vi "Main.vi"() -> ()   [LabVIEW 2023]
panel:
  out "Result":dbl
  in  "Divide":bool
  in  "Multiply":bool
  in  "Subtract":bool
  in  "Add":bool
  in  "Operand 2":dbl
  in  "Operand 1":dbl
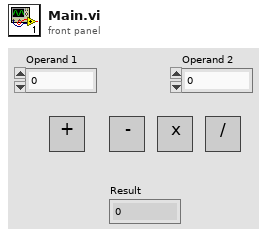
[diagram p1: front panel]
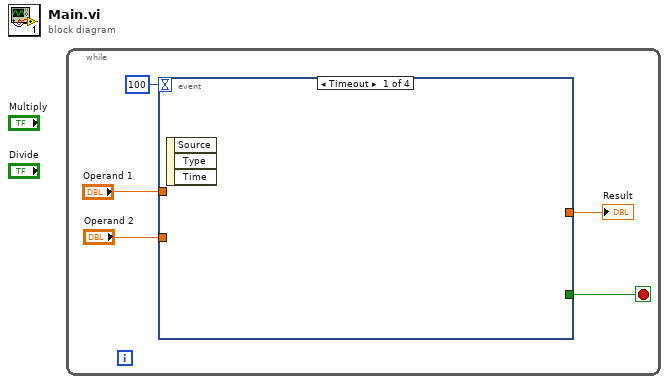
[diagram p0: block diagram]
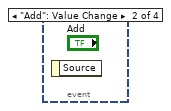
[diagram p2: hidden frame]
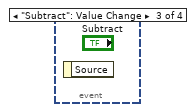
[diagram p3: hidden frame]
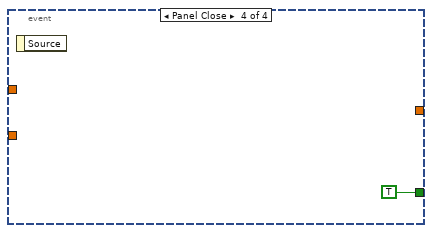
[diagram p4: hidden frame]
diagram:
  n1 = while {
    stop <- w1 stop-if-true
    n2 = event shown="[0] Timeout" {
      selector: _ -> [_ _ _ _]
      dyn-events: _ -> [_ _ _ _]
      timeout: 100 -> [_ _ _ _]
      tunnel: "Operand 1" -> [_ _ _ _]
      tunnel: "Operand 2" -> [_ _ _ _]
      tunnel: [_ _ _ _] -> w2
      tunnel: [_ _ _ TRUE] -> w1
      event Timeout {
        n3 = event-data() -> ()  [unwired: 1 in, 3 out]
      }
      event "Add": Value Change {
        n4 = event-data() -> ()  [unwired: 1 in, 1 out]
      }
      event "Subtract": Value Change {
        n5 = event-data() -> ()  [unwired: 1 in, 1 out]
      }
      event Panel Close {
        n6 = event-data() -> ()  [unwired: 1 in, 1 out]
      }
    }
    "Result" <- w2
  }
